vi "read_calibration.vi"(8 "error in":errorcluster, 11 "Calibration file name":path=path "C:/Documents and Settings/ram/My Documents/work/asap/labview/calibration.dat") -> (0 "error out":errorcluster, 2 "Calibration data":T1)   [LabVIEW 2012]
uses:
  initialization/asap_calibration.ctl
  <vilib>/Analysis/Matrix/Datatypes/RealMatrix.ctl
  utilities/labview/read_matrix_reshape_3D.vi
  utilities/labview/read_matrix_reshape_4D.vi
  <vilib>/Analysis/Matrix/NI_Matrix.lvlib
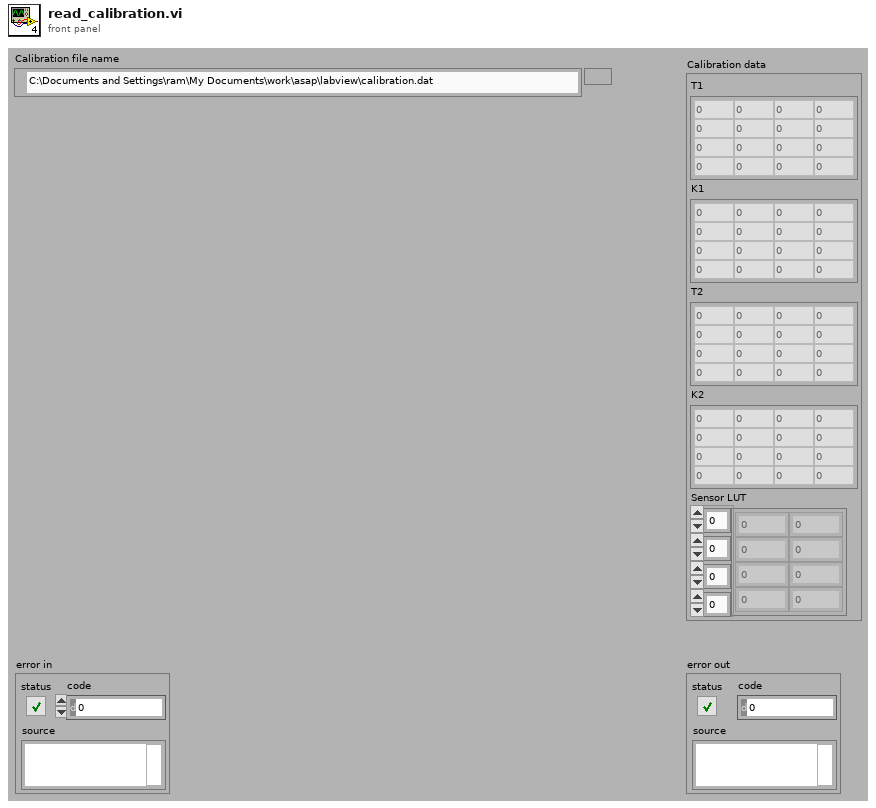
[diagram p1: front panel]
types:
  T1 = typedef "asap_calibration.ctl" = cluster{"T1":T2, "K1":T2, "T2":T2, "K2":T2, "Sensor LUT":sgl[][][][]}
  T2 = typedef "NI_Matrix.lvlib/RealMatrix.ctl" = dbl[][]
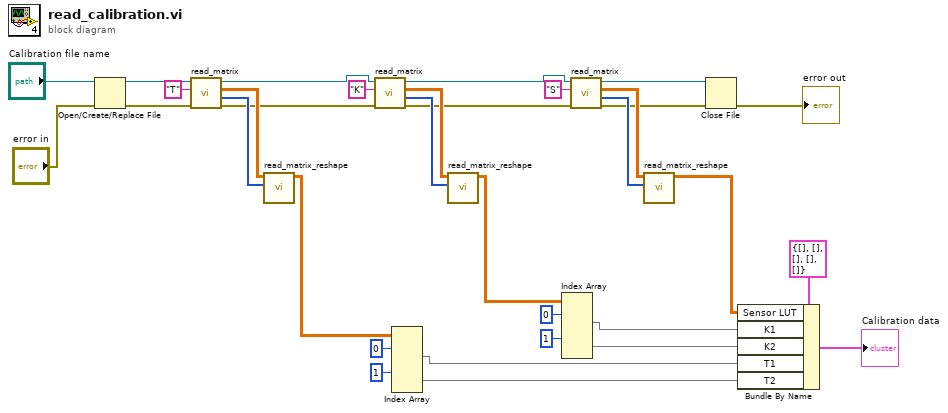
[diagram p0: block diagram]
diagram:
  n1 = Open/Create/Replace File(file path (use dialog)="Calibration file name", error in="error in") -> (refnum out=w32:refnum<file>, error out=w30:errorcluster)  [unwired: 4 in, 1 out]
  n2 = call "read_matrix.vi"("error in"=w30, "Entry name"="T", "file refnum"=w32) -> ("error out"=w22:errorcluster, "Dimensions"=w27:i32[], "Result"=w28:dbl[][], "refnum out"=w23:refnum<file>)  [unwired: 4 in, 1 out]
  n3 = call-poly "read_matrix_reshape.vi"("Dimensions"=w27, "Result in"=w28) -> ("Result out"=w6:dbl[][][])  [unwired: 9 in]
  n4 = call "read_matrix.vi"("error in"=w22, "Entry name"="K", "file refnum"=w23) -> ("error out"=w17:errorcluster, "Dimensions"=w26:i32[], "Result"=w25:dbl[][], "refnum out"=w18:refnum<file>)  [unwired: 4 in, 1 out]
  n5 = Index Array(array=w6, index (dim 0) #1=0 ("index (page)"), index (dim 0) #2=1 ("index (page)")) -> (element #1=w5:dbl[][], element #2=w4:dbl[][])  [unwired: 4 in]
  n6 = call-poly "read_matrix_reshape.vi"("Dimensions"=w26, "Result in"=w25) -> ("Result out"=w13:dbl[][][])  [unwired: 9 in]
  n7 = Index Array(array=w13, index (dim 0) #1=0 ("index (page)"), index (dim 0) #2=1 ("index (page)")) -> (element #1=w10:dbl[][], element #2=w9:dbl[][])  [unwired: 4 in]
  n8 = call "read_matrix.vi"("error in"=w17, "Entry name"="S", "file refnum"=w18) -> ("error out"=w2:errorcluster, "Dimensions"=w19:i32[], "Result"=w20:dbl[][], "refnum out"=w3:refnum<file>)  [unwired: 4 in, 1 out]
  n9 = call-poly "read_matrix_reshape.vi"("Dimensions"=w19, "Result in"=w20) -> ("Result out"=w14:dbl[][][][])  [unwired: 9 in]
  n10 = Close File(refnum=w3, error in=w2) -> (error out=→"error out":errorcluster)  [unwired: 1 out]
  n11 = Bundle By Name(cluster=T1 {"T1"=[], "K1"=[], "T2"=[], "K2"=[], "Sensor LUT"=[]} ("Calibration data"), "Sensor LUT"=w14, "K1"=w10, "K2"=w9, "T1"=w5, "T2"=w4) -> (→"Calibration data":T1)
